vi "Keithley 622x Set Sweep.vi"(6 "Step":dbl=0.0001 format="%#_6p", 7 "Delay":dbl=0.0001 format="%#_6p", 8 "error in":errorcluster, 9 "End":dbl=0.001 format="%#_6p", 10 "Start":dbl=-0.001 format="%#_6p", 11 "VISA resource name":refnum<visa-resource-name>) -> (0 "error out":errorcluster, 3 "VISA resource name out":refnum<visa-resource-name>)   [LabVIEW 2021]
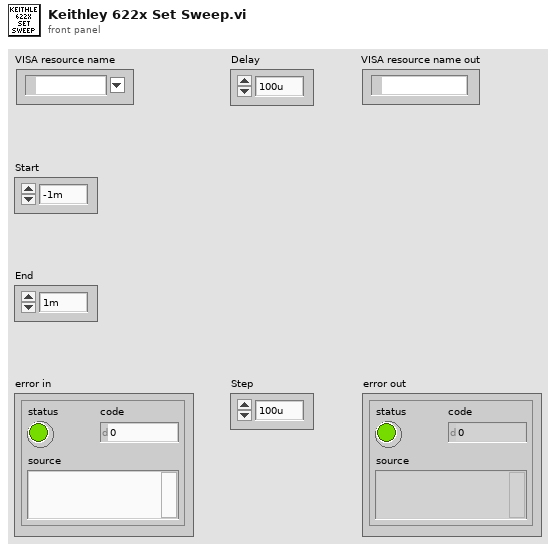
[diagram p1: front panel]
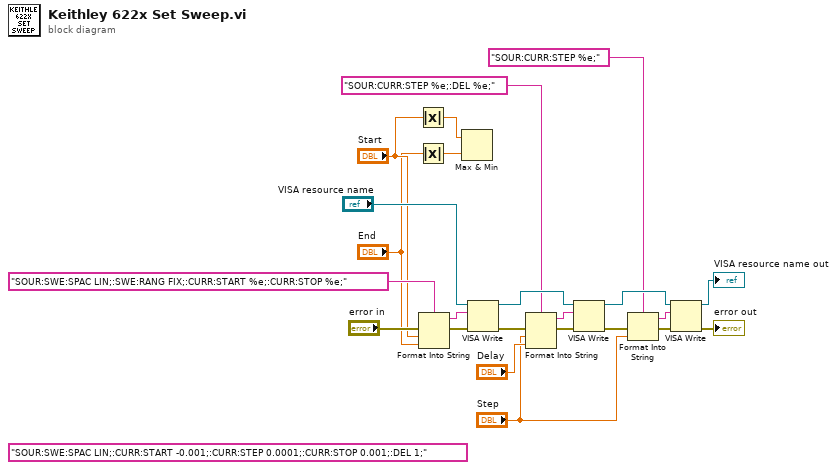
[diagram p0: block diagram]
diagram:
  (unwired) "SOUR:SWE:SPAC LIN;:CURR:START -0.001;:CURR:STEP 0.0001;:CURR:STOP 0.001;:DEL 1;"
  n1 = Absolute Value(x="Start") -> (abs(x)=w18:dbl)
  n2 = Absolute Value(x="End") -> (abs(x)=w17:dbl)
  n3 = Format Into String(format string="SOUR:SWE:SPAC LIN;:SWE:RANG FIX;:CURR:START %e;:CURR:STOP %e;", error in="error in", "Start", "End") -> (resulting string=w19:string, error out=w23:errorcluster)  [unwired: 1 in]
  n4 = Max & Min(x=w18, y=w17) -> ()  [unwired: 2 out]
  n5 = VISA Write(VISA resource name="VISA resource name", write buffer=w19, error in (no error)=w23) -> (VISA resource name out=w14:refnum<visa-resource-name>, error out=w13:errorcluster)  [unwired: 1 out]
  n6 = Format Into String(format string="SOUR:CURR:STEP %e;:DEL %e;", error in=w13, "Step", "Delay") -> (resulting string=w9:string, error out=w12:errorcluster)  [unwired: 1 in]
  n7 = VISA Write(VISA resource name=w14, write buffer=w9, error in (no error)=w12) -> (VISA resource name out=w7:refnum<visa-resource-name>, error out=w5:errorcluster)  [unwired: 1 out]
  n8 = Format Into String(format string="SOUR:CURR:STEP %e;", error in=w5, "Step") -> (resulting string=w3:string, error out=w4:errorcluster)  [unwired: 1 in]
  n9 = VISA Write(VISA resource name=w7, write buffer=w3, error in (no error)=w4) -> (VISA resource name out=→"VISA resource name out":refnum<visa-resource-name>, error out=→"error out":errorcluster)  [unwired: 1 out]
